vi "New TDMS Channel.vi"(8 "error in (no error)":errorcluster, 11 "TDMS Channel":T1) -> (0 "error out":errorcluster, 3 "TdmsChannel Ref":T3)   [LabVIEW 2020, in "NI_VS Data Logging API.lvlib"]
doc: "Creates a TdmsChannel object based on the settings in the <b>TDMS Channel</b> input."
uses:
  <vilib>/NI VeriStand/Execution/DataLogging/NI_VS Data Logging API.lvlib
  <vilib>/NI VeriStand/Execution/DataLogging/TdmsChannel Ref.ctl
  NationalInstruments.VeriStand.ClientAPI
  <vilib>/NI VeriStand/Execution/DataLogging/TDMS Channel.ctl
  <vilib>/NI VeriStand/Execution/DataLogging/TDMS Property.ctl
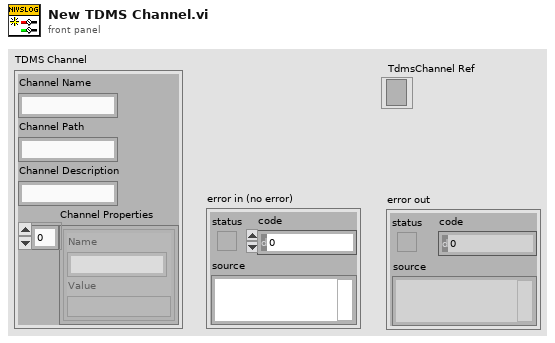
[diagram p1: front panel]
types:
  T1 = typedef "NI_VS Data Logging API.lvlib/TDMS Channel.ctl" = cluster{"Channel Name":string, "Channel Path":string, "Channel Description":string, "Channel Properties":T2[]}
  T2 = typedef "NI_VS Data Logging API.lvlib/TDMS Property.ctl" = cluster{"Name":string, "Value":variant}
  T3 = typedef "NI_VS Data Logging API.lvlib/TdmsChannel Ref.ctl" = refnum<k24>
  T4 = typedef "NI_VS Data Logging API.lvlib/TdmsProperty Ref.ctl" = refnum<k24>
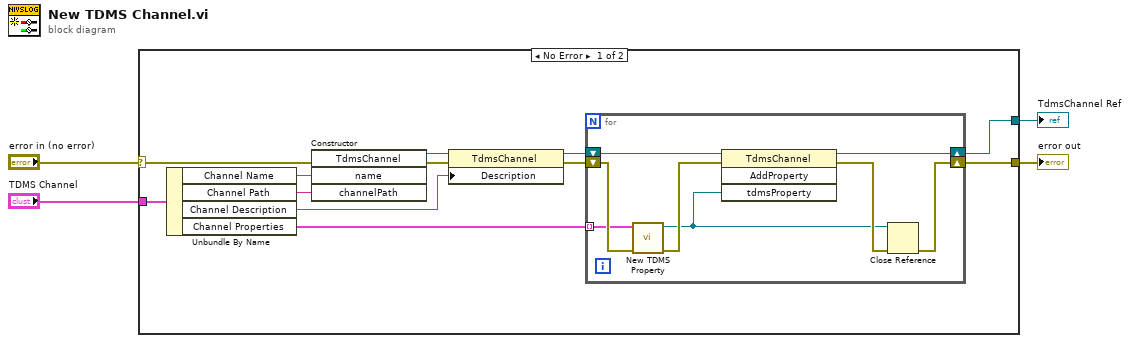
[diagram p0: block diagram]
diagram:
  n1 = case shown="No Error" "error in (no error)" {
    selector: "error in (no error)" -> [w9 w25]
    tunnel: "TDMS Channel" -> [w8 _]
    tunnel: [w6 _] -> w2
    tunnel: [w5 w25] -> w1
    frame No Error {
      n2 = Unbundle By Name(w8) -> ("Channel Name"=w16:string, "Channel Path"=w7:string, "Channel Description"=w13:string, "Channel Properties"=w10:T2[])
      n3 = constructor class="TdmsChannel"(error in=w9, "name"=w16, "channelPath"=w7) -> (reference out=w15:refnum<k24>, error out=w14:errorcluster)  [unwired: 2 in, 3 out]
      n4 = property class="TdmsChannel"(reference=w15, error in=w14, "Description"=w13) -> (reference out=w12:refnum<k24>, error out=w11:errorcluster)
      n5 = for {
        tunnel: w10 -> [w20] mode=indexing
        shift-right: [w21] -> w6
        shift-left: w12 -> [w22]
        shift-right: [w17] -> w5
        shift-left: w11 -> [w23]
        n6 = call <vilib>:"New TDMS Property.vi"("error in (no error)"=w23, "TDMS Property"=w20) -> ("error out"=w24:errorcluster, "TDMSProperty Ref"=w18:T4)  [unwired: 8 in]
        n7 = invoke class="TdmsChannel" method="AddProperty"(reference=w22, error in=w24, "tdmsProperty"=w18) -> (reference out=w21:refnum<k24>, error out=w19:errorcluster)  [unwired: 1 in, 2 out]
        n8 = Close Reference(reference=w18, error in (no error)=w19) -> (error out=w17:errorcluster)
      }
    }
    frame Error {
    }
  }
  "TdmsChannel Ref" <- w2
  "error out" <- w1
